vi "HoloPy_volume_and_focus.vi"(8 "error in (no error)":errorcluster, 11 "Refnum in":refnum<k35>) -> (0 "error out":errorcluster, 2 "return value":string, 3 "Refnum out":refnum<k35>)   [LabVIEW 2025, in "holoTracker.lvlib"]
uses:
  holoTracker.lvlib
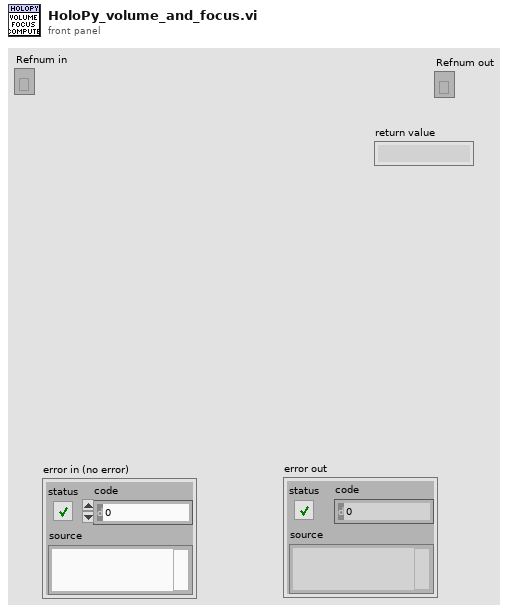
[diagram p1: front panel]
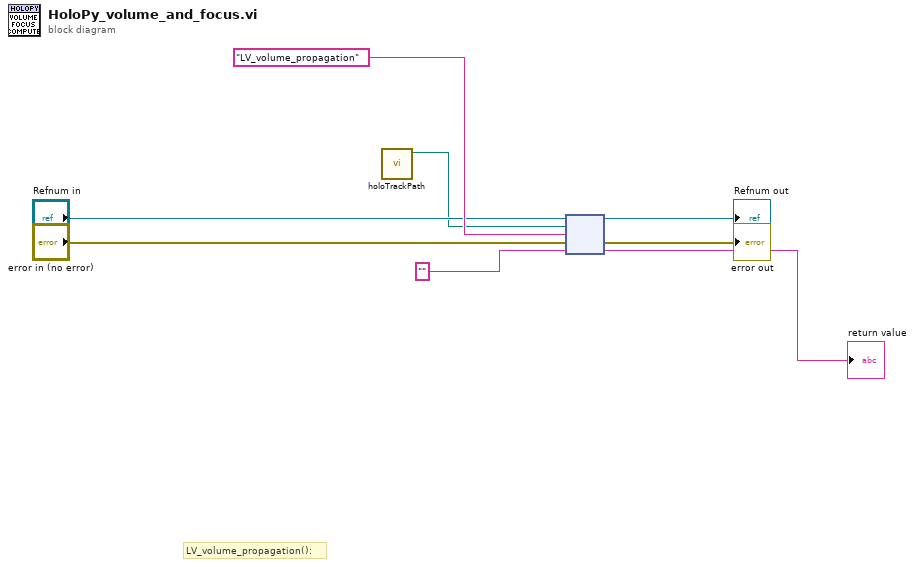
[diagram p0: block diagram]
diagram:
  # "LV_volume_propagation():"
  n1 = call "holoTrackPath.vi"() -> ("appended path"=w1:path)  [unwired: 11 in]
  n2 = node("Refnum in", w1, "LV_volume_propagation" ("function name"), "error in (no error)", "") -> (→"Refnum out":refnum<k35>, →"error out":errorcluster, →"return value":string)  [unwired: 2 out]
